vi "Main.vi"() -> ()   [LabVIEW 2022 SP3]
panel:
  in  "stop send":bool
  in  "stop enqueue":bool
  out "response":string
  in  "data source rid":string="ri.nominal.cerulean-staging.datasource.90dc3651-dded-465d-8885-370b5bc13cc4"
  in  "token":string
  out "exit error out":errorcluster
  out "send error out":errorcluster
  out "enqueue error out":errorcluster
  # "User Inputs"
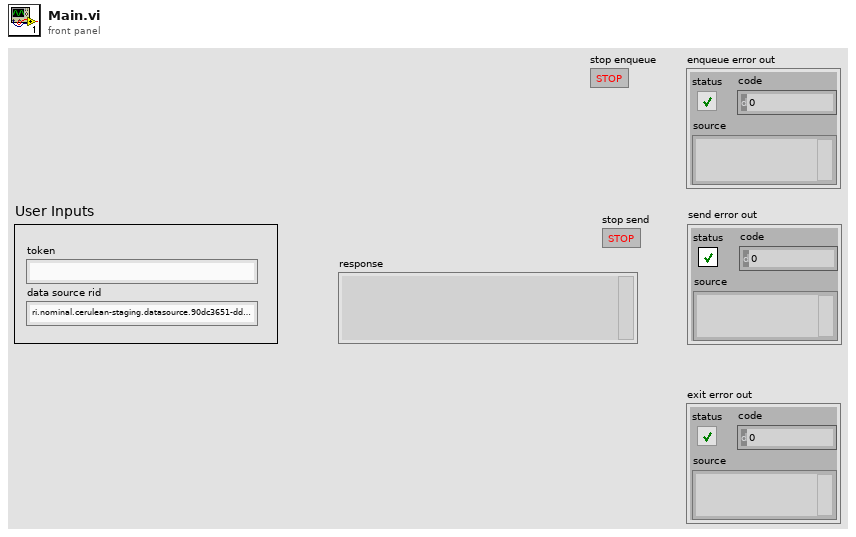
[diagram p1: front panel]
types:
  T1 = typedef "LabVIEWHTTPClient.lvlib/ClientHandle.ctl" = refnum<k1>
  T2 = cluster{"data source rid":string, "queue out":refnum<queue>}
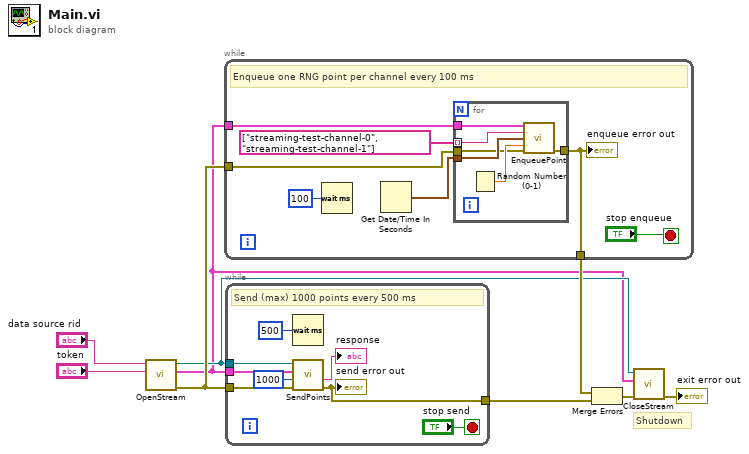
[diagram p0: block diagram]
diagram:
  # "Shutdown"
  n1 = call "OpenStream.vi"("data source rid"="data source rid", "token"="token") -> ("client handle out"=w4:T1, "queue out"=w3:T2, "error out"=w9:errorcluster)  [unwired: 6 in]
  n2 = while {
    tunnel: w3 -> [w14]
    tunnel: w9 -> [w12]
    tunnel: [w11] -> w6
    stop <- "stop enqueue" stop-if-true
    # "Enqueue one RNG point per channel every 100 ms"
    n3 = Wait (ms)(milliseconds to wait=u32 100) -> ()  [unwired: 1 out]
    n4 = Get Date/Time In Seconds() -> (seconds since 1Jan1904=w13:timestamp)
    n5 = for {
      tunnel: string[] ["streaming-test-channel-0", "streaming-test-channel-1"] ("channel") -> [w22] mode=indexing
      tunnel: w14 -> [w21]
      tunnel: w13 -> [w19]
      tunnel: w12 -> [w18]
      tunnel: [w17] -> w11
      n6 = Random Number (0-1)() -> (number: 0 to 1=w20:dbl)
      n7 = call "EnqueuePoint.vi"("queue in"=w21, "channel"=w22, "time"=w19, "value"=w20, "error in (no error)"=w18) -> ("error out"=w17:errorcluster)  [unwired: 8 in, 2 out]
    }
    "enqueue error out" <- w11
  }
  n8 = while {
    tunnel: w3 -> [w29]
    tunnel: w9 -> [w28]
    tunnel: w4 -> [w27]
    tunnel: [w25] -> w5
    stop <- "stop send" stop-if-true
    # "Send (max) 1000 points every 500 ms"
    n9 = Wait (ms)(milliseconds to wait=u32 500) -> ()  [unwired: 1 out]
    n10 = call "SendPoints.vi"("error in (no error)"=w28, "max points to send"=1000, "queue in"=w29, "client handle"=w27) -> ("error out"=w25:errorcluster, "response"=→"response":string)  [unwired: 4 in, 2 out]
    "send error out" <- w25
  }
  n11 = Merge Errors(w6, w5) -> (w7:errorcluster)
  n12 = call "CloseStream.vi"("client handle"=w4, "queue in"=w3, "error in (no error)"=w7) -> ("error out"=→"exit error out":errorcluster)  [unwired: 6 in, 1 out]
